vi "Configure Marker Frequency.vi"(8 "error in (no error)":errorcluster, 9 "Marker Number (1)":u32=1 min=1, 10 "Marker Frequency [Hz]":dbl, 11 "MXA in":refnum<class "MXA.lvclass">) -> (0 "error out":errorcluster, 3 "MXA out":refnum<class "MXA.lvclass">)   [LabVIEW 2020, in "MXA.lvclass"]
uses:
  MXA.lvclass
  C:/Sandbox/RF Bench/Source Code/WiSpry Test Framework/Instruments/Instrument.lvclass
  Instrument.lvclass/Instrument.ctl
  Instrument.lvclass
  <instrlib>/Agilent MXA Series/Agilent MXA Series.lvlib
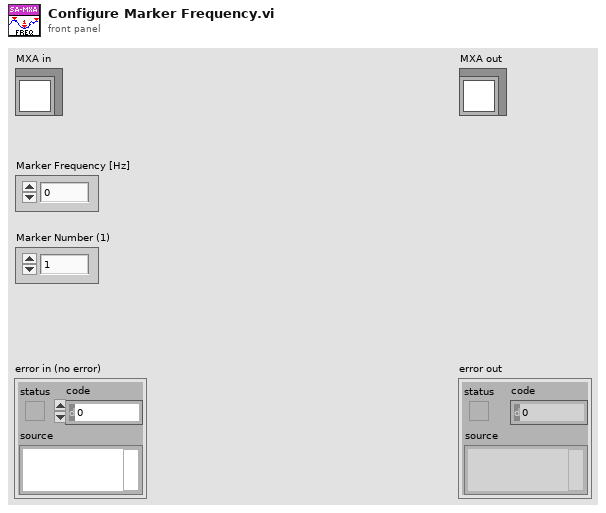
[diagram p1: front panel]
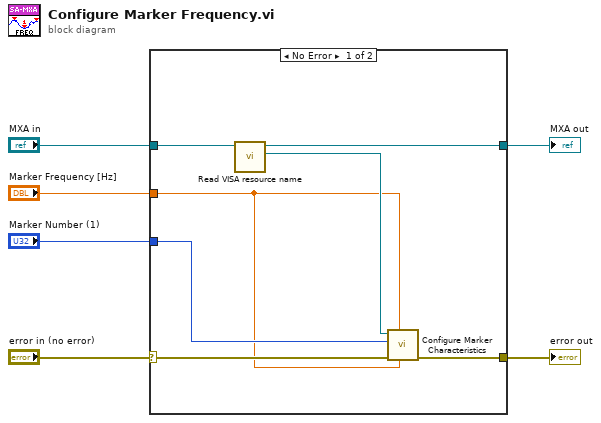
[diagram p0: block diagram]
diagram:
  n1 = case shown="No Error" "error in (no error)" {
    selector: "error in (no error)" -> [w10 w15]
    tunnel: "MXA in" -> [w13 w14]
    tunnel: [w9 w15] -> w5
    tunnel: [w12 w14] -> w4
    tunnel: "Marker Number (1)" -> [w8 _]
    tunnel: "Marker Frequency [Hz]" -> [w7 _]
    frame No Error {
      n2 = call "Read VISA resource name.vi"("Instrument in"=w13) -> ("VISA resource name"=w11:refnum<visa-resource-name>, "Instrument out"=w12:refnum<class "MXA.lvclass">)  [unwired: 9 in]
      n3 = call <instrlib>:"Configure Marker Characteristics.vi"("Band Right Edge Frequency (0 Hz)"=w7, "Band Left Edge Frequency (0 Hz)"=w7, "error in (no error)"=w10, "Active Marker (1: Marker1)"=w8, "VISA resource name"=w11) -> ("error out"=w9:errorcluster)  [unwired: 5 in, 1 out]
    }
    frame Error {
    }
  }
  "error out" <- w5
  "MXA out" <- w4
